vi "PS35_KD.vi"(0 "Axis number":i32=1 min=1 max=3, 1 "Control unit ID":i32=1 min=1 max=10, 2 "Value-In":i32=150 min=0 max=32767, 3 "error in (no error)":errorcluster, 5 "function":bool) -> (7 "Value-Out":i32, 9 "error out":errorcluster)   [LabVIEW 2020]
doc: "PS35_KD.vi, created: 05.03.2009 alex; last change: 22.10.2019 alex;\n\n<B>FUNCTIONS:</B> \n\n<B>Read:</B> FALSE: read D parameter of the PID regulator for an axis.\n<B>Write:</B> TRUE: set D parameter of the PID regulator for an axis.\nThis is valid only for the axes with encoder (DC-Brush, Stepper Closed Loop). \n----------------------------------------------------------------------------------------\n<B>INPUT:</B>\n[TF] <B>function:</B> function selector. (Read, Write)\n[I32] <B>Control unit ID:</B> control unit index. (Default=1, Range=1...10)\n[I32] <B>Axis number:</B> axis number. (Default=1, Range=1...3)\n[I32] <B>Value-In:</B> D parameter. (only for Write: Default=150, Range=0…32767)\n[CLU] <B>error in</B>\n----------------------------------------------------------------------------------------\n<B>OUTPUT:</B>\n[I32] <B>Value-Out:</B> D parameter. (for Write: Value-Out=Value-In)\n[CLU] <B>error out</B>\n----------------------------------------------------------------------------------------\n<B>SUB-VIs:</B>\nPS35_GetReadError.vi\n----------------------------------------------------------------------------------------\n<B>EXT-Calls:</B>\nps35.dll (V2.01)\n----------------------------------------------------------------------------------------"
uses:
  ps35.dll
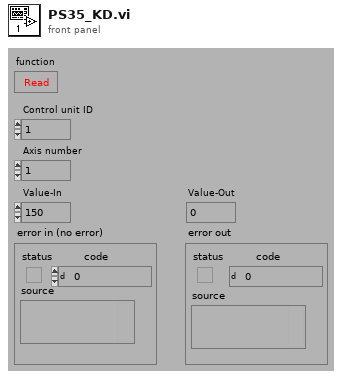
[diagram p1: front panel]
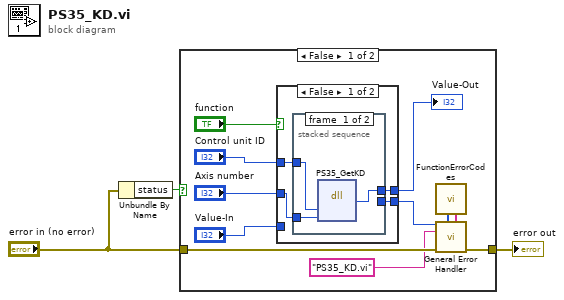
[diagram p0: block diagram]
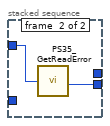
[diagram p2: hidden frame]
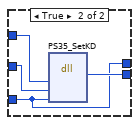
[diagram p3: hidden frame]
diagram:
  n1 = Unbundle By Name("error in (no error)") -> ("status"=w1:bool)
  n2 = case shown="False" w1 {
    tunnel: "error in (no error)" -> [w14 w28]
    tunnel: [w13 w28] -> w3
    frame False {
      n3 = case shown="False" "function" {
        tunnel: "Control unit ID" -> [w17 w26]
        tunnel: [w18 w27] -> w10
        tunnel: "Value-In" -> [_ w24]
        tunnel: [w16 w24] -> w8
        tunnel: "Axis number" -> [w15 w25]
        frame False {
          n4 = stacked-sequence {
            tunnel: [_ w23] -> w18
            tunnel: w17 -> [w21 w22]
            tunnel: [w20 _] -> w16
            tunnel: w15 -> [w19 _]
            frame #0 {
              n5 = dll-call lib="C:/GEECS/Developers Version/source/Device Drivers/OwiSoft/OWISoftOEM/ps35/labview/lv82/ps35.dll" fn="PS35_GetKD" label="PS35_\nGetKD"("Index"=w21, "AxisNr"=w19) -> ("Rückgabetyp"=w20:i32)  [unwired: 5 in, 2 out]
            }
            frame #1 {
              n6 = call "PS35_GetReadError.vi"("Control unit ID"=w22) -> ("Read error"=w23:i32)
            }
          }
        }
        frame True {
          n7 = dll-call lib="C:/GEECS/Developers Version/source/Device Drivers/OwiSoft/OWISoftOEM/ps35/labview/lv82/ps35.dll" fn="PS35_SetKD" label="PS35_\nSetKD"("Index"=w26, "AxisNr"=w25, "Value"=w24) -> ("Rückgabetyp"=w27:i32)  [unwired: 6 in, 2 out]
        }
      }
      "Value-Out" <- w8
      n8 = call "FunctionErrorCodes.vi"() -> ("[user-defined codes]"=w5:i32[], "[user-defined descriptions]"=w4:string[])  [unwired: 8 in]
      n9 = call <vilib>:"General Error Handler.vi"("[error code] (0)"=w10, "[user-defined codes]"=w5, "[user-defined descriptions]"=w4, "[error source] (\" \")"="PS35_KD.vi" ("[error source] (\" \")"), "error in (no error)"=w14) -> ("error out"=w13:errorcluster)  [unwired: 6 in, 4 out]
    }
    frame True {
    }
  }
  "error out" <- w3
